vi "get NodePath for traverse.vi"(8 "error in (no error)":errorcluster caption="错误输入（无错误）", 10 "Data in":string[](array[string]), 11 "Class in":refnum<class "PanelLinkNode.lvclass">) -> (0 "error out":errorcluster caption="错误输出", 2 "Data out":string[](array[string]), 3 "Class out":refnum<class "PanelLinkNode.lvclass">)   [LabVIEW 2016, in "PanelLinkNode.lvclass"]
uses:
  PanelLinkNode.lvclass
  PanelLinkNode.lvclass/PanelLinkNode.ctl
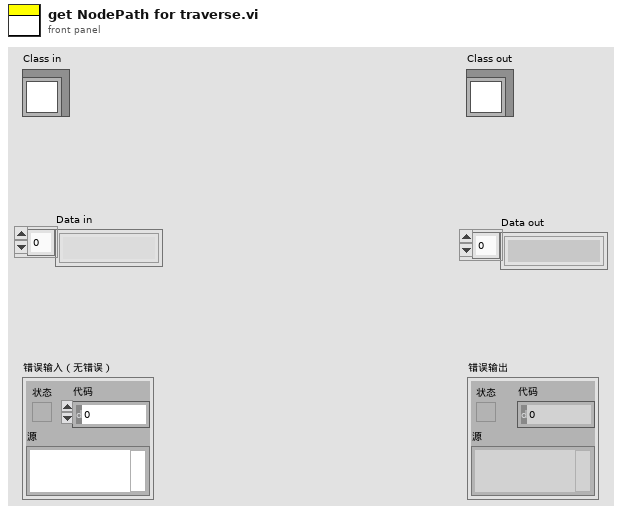
[diagram p1: front panel]
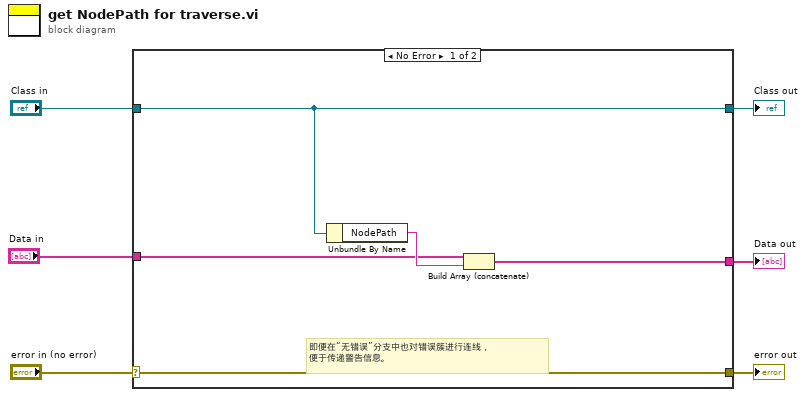
[diagram p0: block diagram]
diagram:
  n1 = case shown="No Error" "error in (no error)" {
    selector: "error in (no error)" -> [w8 w14]
    tunnel: [w8 w14] -> w5
    tunnel: [w10 w13] -> w3
    tunnel: "Class in" -> [w10 w13]
    tunnel: "Data in" -> [w9 w12]
    tunnel: [w7 w12] -> w1
    frame No Error {
      # "即便在“无错误”分支中也对错误簇进行连线，\n便于传递警告信息。"
      n2 = Unbundle By Name(w10) -> ("NodePath"=w11:string)
      n3 = Build Array (concatenate)(w9, w11) -> (w7:string[])
    }
    frame Error {
    }
  }
  "error out" <- w5
  "Class out" <- w3
  "Data out" <- w1
